vi "Write End Time.vi"(8 "error in (no error)":errorcluster, 10 "End Time":timestamp format="%<%x %.3X>T", 11 "Time Entries in":refnum<class "Time Entries.lvclass">) -> (0 "error out":errorcluster, 3 "Time Entries out":refnum<class "Time Entries.lvclass">)   [LabVIEW 2020, in "Time Entries.lvclass"]
uses:
  Time Entries.lvclass
  Time Entries.lvclass/Time Entries.ctl
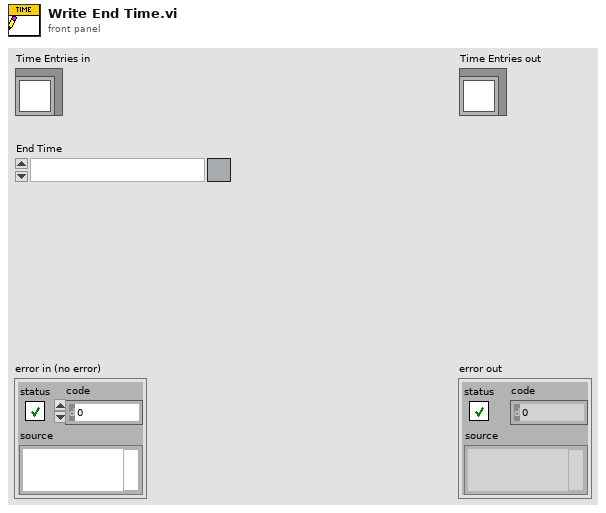
[diagram p1: front panel]
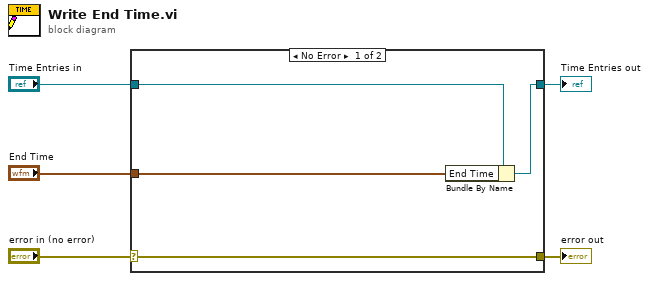
[diagram p0: block diagram]
diagram:
  n1 = case shown="No Error" "error in (no error)" {
    selector: "error in (no error)" -> [w9 w10]
    tunnel: [w9 w10] -> w4
    tunnel: [w7 w11] -> w2
    tunnel: "Time Entries in" -> [w8 w11]
    tunnel: "End Time" -> [w6 _]
    frame No Error {
      n2 = Bundle By Name(cluster=w8, "End Time"=w6) -> (w7:refnum<class "Time Entries.lvclass">)
    }
    frame Error {
    }
  }
  "error out" <- w4
  "Time Entries out" <- w2
